vi "Write.vi"(8 "error in":errorcluster, 10 "CAN Messages":refnum<class "CAN Message.lvclass">[](array[class]), 11 "PCAN in":refnum<class "Messaging Manager Actor.lvclass">) -> (0 "error out":errorcluster, 3 "PCAN out":refnum<class "Messaging Manager Actor.lvclass">)   [LabVIEW 2024, in "PCAN.lvlib" / "Messaging Manager Actor.lvlib" / "Messaging Manager Actor.lvclass"]
uses:
  Messaging Manager Actor.lvclass
  CAN Message/CAN Message.lvclass
  Messaging Manager Actor.lvclass/Messaging Manager Actor.ctl
  <instrlib>/KDI Digital Instrumentation/API_for_PCAN_BASIC_FD/Error language selector.ctl
  <instrlib>/KDI Digital Instrumentation/API_for_PCAN_BASIC_FD/CAN MSG Cluster.ctl
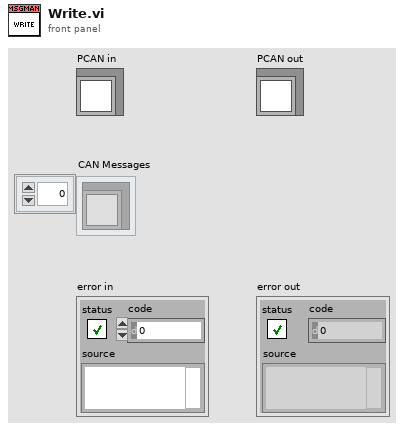
[diagram p1: front panel]
types:
  T1 = typedef "TPCANHandle.ctl" = enum16{"PCAN_NONEBUS  0x000", "PCAN_ISABUS1  0x21", "PCAN_ISABUS2  0x22", "PCAN_ISABUS3  0x23", "PCAN_ISABUS4  0x24", "PCAN_ISABUS5  0x25", "PCAN_ISABUS6  0x26", "PCAN_ISABUS7  0x27", "PCAN_ISABUS8  0x28", "PCAN_DNGBUS1  0x31", "PCAN_PCIBUS1  0x41", "PCAN_PCIBUS1  0x42", "PCAN_PCIBUS1  0x43", "PCAN_PCIBUS1  0x44", "PCAN_PCIBUS1  0x45", "PCAN_PCIBUS1  0x46", "PCAN_PCIBUS1  0x47", "PCAN_PCIBUS1  0x48", "PCAN_PCIBUS1  0x409", "PCAN_PCIBUS1  0x40A", "PCAN_PCIBUS1  0x40B", "PCAN_PCIBUS1  0x40C", "PCAN_PCIBUS1  0x40D", "PCAN_PCIBUS1  0x40E", "PCAN_PCIBUS1  0x40F", "PCAN_PCIBUS1  0x410", "PCAN_USBBUS1  0x51", "PCAN_USBBUS2  0x52", "PCAN_USBBUS3  0x53", "PCAN_USBBUS4  0x54", "PCAN_USBBUS5  0x55", "PCAN_USBBUS6  0x56", "PCAN_USBBUS7  0x57", "PCAN_USBBUS8  0x58", "PCAN_USBBUS9  0x509", "PCAN_USBBUS10  0x50A", "PCAN_USBBUS11  0x50B", "PCAN_USBBUS12  0x50C", "PCAN_USBBUS13  0x50D", "PCAN_USBBUS14  0x50E", "PCAN_USBBUS15  0x50F", "PCAN_USBBUS16  0x510", "PCAN_PCCBUS1  0x61", "PCAN_PCCBUS2  0x62", "PCAN_LANBUS1  0x801", "PCAN_LANBUS2  0x802", "PCAN_LANBUS3  0x803", "PCAN_LANBUS4  0x804", "PCAN_LANBUS5  0x805", "PCAN_LANBUS6  0x806", "PCAN_LANBUS7  0x807", "PCAN_LANBUS8  0x808", "PCAN_LANBUS9  0x809", "PCAN_LANBUS10  0x80A", "PCAN_LANBUS11  0x80B", "PCAN_LANBUS12  0x80C", "PCAN_LANBUS13  0x80D", "PCAN_LANBUS14  0x80E", "PCAN_LANBUS15  0x80F", "PCAN_LANBUS16  0x810"}
  T2 = typedef "CAN MSG Cluster.ctl" = cluster{"ID":u32, "MSG type":u8, "DLC":u8, "DATA":u8[]}
  T3 = typedef "Error language selector.ctl" = u16
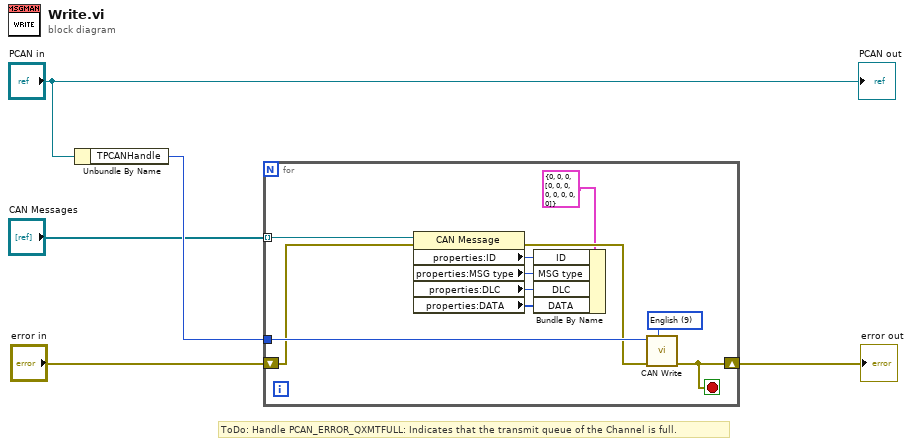
[diagram p0: block diagram]
diagram:
  # "ToDo: Handle PCAN_ERROR_QXMTFULL: Indicates that the transmit queue of the Channel is full."
  n1 = Unbundle By Name("PCAN in") -> ("TPCANHandle"=w5:T1)
  n2 = for {
    tunnel: w5 -> [w16]
    shift-right: [w9] -> w4
    shift-left: "error in" -> [w11]
    tunnel: "CAN Messages" -> [w7] mode=indexing
    stop <- w9 stop-if-true
    w8 = T3 9 items=["System dependent", "Not available", "Not available", "Not available", "Not available", "Not available", "Not available", "Deutsch", "Not available", "English", "Español", "Not available", "Français", "Not available", "Not available", "Not available", "Italiano"] ("Language")
    n3 = property class="CAN Message"(reference=w7, error in=w11) -> (error out=w10:errorcluster, "properties:ID"=w12:u32, "properties:MSG type"=w13:u8, "properties:DLC"=w14:u8, "properties:DATA"=w15:u8[])  [unwired: 1 out]
    n4 = Bundle By Name(cluster=T2 {"ID"=0, "MSG type"=0, "DLC"=0, "DATA"=[0, 0, 0, 0, 0, 0, 0, 0]} ("CAN_Message"), "ID"=w12, "MSG type"=w13, "DLC"=w14, "DATA"=w15) -> ()  [unwired: 1 out]
    n5 = call <instrlib>:"CAN Write.vi"("Language"=w8, "error in (no error)"=w10, "TPCANHandle"=w16) -> ("error out"=w9:errorcluster)  [unwired: 7 in, 1 out]
  }
  "error out" <- w4
  "PCAN out" <- "PCAN in"
